vi "VI Set Inline.vi"(8 "error in (no error)":errorcluster, 10 "Inline VI":bool, 11 "vi ref in":refnum<vi>) -> (0 "error out":errorcluster, 3 "vi ref out":refnum<vi>)   [LabVIEW 2019, in "Build Automation.lvlib"]
uses:
  Build Automation.lvlib
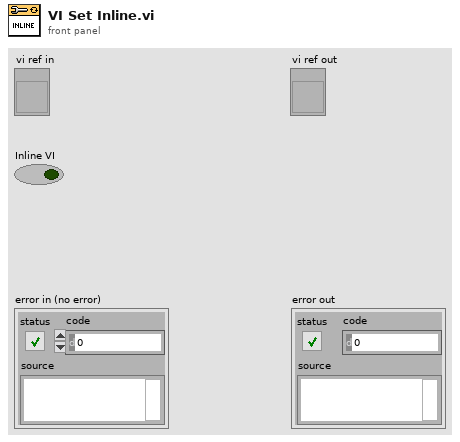
[diagram p1: front panel]
types:
  T1 = enum32{"Bad", "Idle", "Run top level", "Running"}
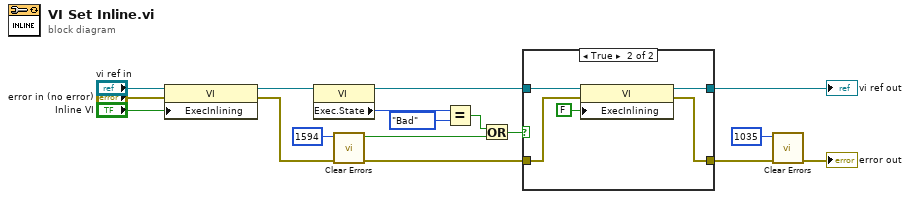
[diagram p0: block diagram]
diagram:
  n1 = property class="VI"(reference="vi ref in", error in="error in (no error)", "ExecInlining"="Inline VI") -> (reference out=w10:refnum<vi>, error out=w12:errorcluster)
  n2 = property class="VI"(reference=w10) -> (reference out=w9:refnum<vi>, "Exec.State"=w8:T1)  [unwired: 1 in, 1 out]
  n3 = call <vilib>:"Clear Errors.vi"("error in (no error)"=w12, "specific error code to clear (0: all)"=1594) -> ("error out"=w1:errorcluster, "specific error cleared?"=w4:bool)  [unwired: 4 in]
  n4 = Equal?(x=w8, y=T1."Bad" ("Execution:State")) -> (x = y?=w5:bool)
  n5 = Or(x=w5, y=w4) -> (x .or. y?=w6:bool)
  n6 = case shown="True" w6 {
    tunnel: w9 -> [w19 w24]
    tunnel: [w19 w23] -> w3
    tunnel: [w18 w22] -> w11
    tunnel: w1 -> [w18 w20]
    frame False {
    }
    frame True {
      n7 = property class="VI"(reference=w24, error in=w20, "ExecInlining"=FALSE ("Execution:Inline SubVI")) -> (reference out=w23:refnum<vi>, error out=w22:errorcluster)
    }
  }
  "vi ref out" <- w3
  n8 = call <vilib>:"Clear Errors.vi"("error in (no error)"=w11, "specific error code to clear (0: all)"=1035) -> ("error out"=→"error out":errorcluster)  [unwired: 4 in, 1 out]
